vi "Thor8000TCPCommunicator.vi"(0 "EthernetConnection":T1={"IPAddress"="192.168.0.100", "Port"=1234, "Timeout [ms]"=250, "HeaderBytes"=0, "DataBytes"=30}, 5 "ErrorIn":errorcluster, 8 "Data2Write":string=":slot 1;:temp:act? ") -> (14 "Header":string, 16 "DataRead":string=":TEMP:ACT 9.51464272E+000\n", 19 "ErrorOut":errorcluster)   [LabVIEW 2012]
uses:
  WVDNewArchitectureUpdate/WVD_Architecture_Update/TypeDefinitions.llb/TypeDef_WavemeterTCPCluster.ctl
  <vilib>/regexp/Match Regular Expression.xnode
panel:
  # "Currnet Settings:\n++addr 10\n++auto 1\n++eoi 0\n++eos 0\n++eot_enable 0\n++eot_char 0\n++mode 1\n++read_tmo_ms 500\n++savecfg 1\n++ver 01.06.06.00"
  # ":slot 1;:temp:act?"
  # ":slot 2;:ild:act?"
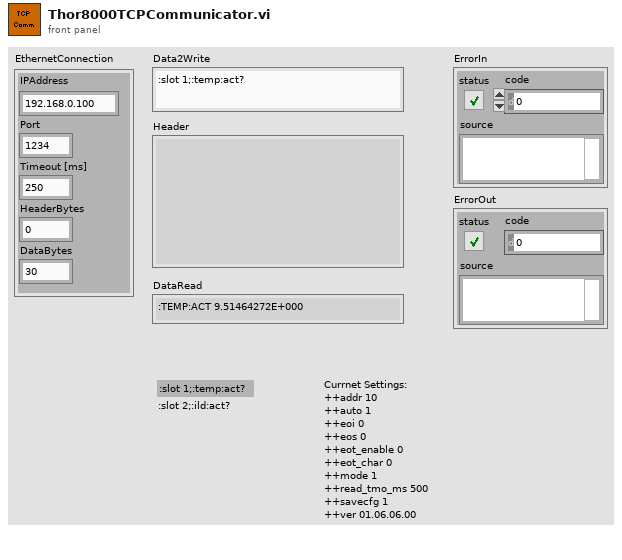
[diagram p1: front panel]
types:
  T1 = typedef "TypeDef_WavemeterTCPCluster.ctl" = cluster{"IPAddress":string, "Port":i16, "Timeout [ms]":i16, "HeaderBytes":i16, "DataBytes":i16}
  T2 = enum16{"Standard", "Buffered", "CRLF", "Immediate"}
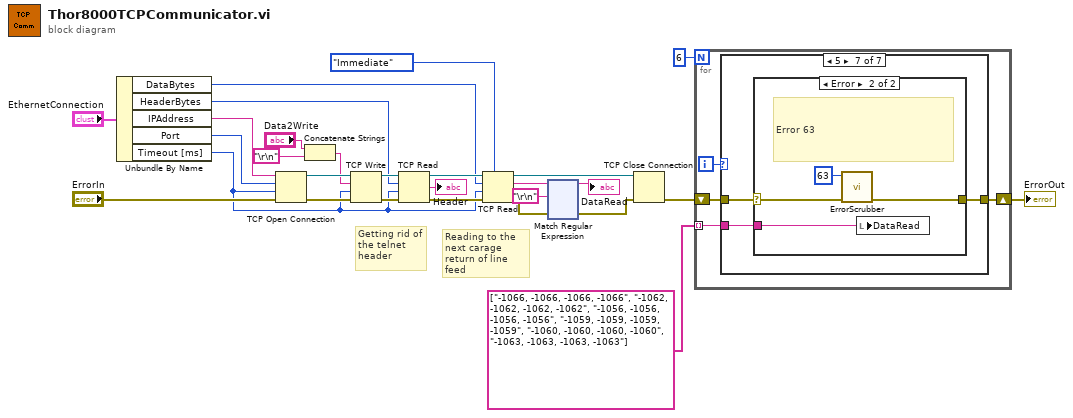
[diagram p0: block diagram]
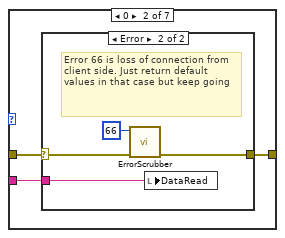
[diagram p3: hidden frame]
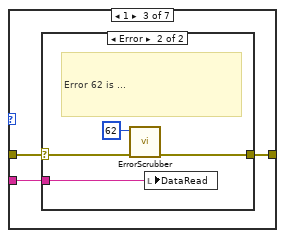
[diagram p5: hidden frame]
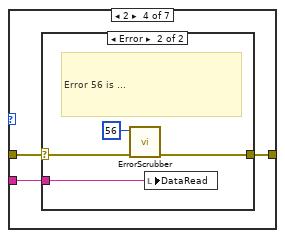
[diagram p7: hidden frame]
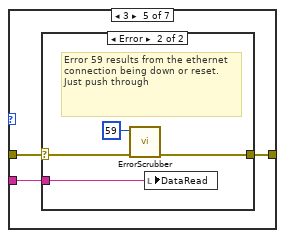
[diagram p9: hidden frame]
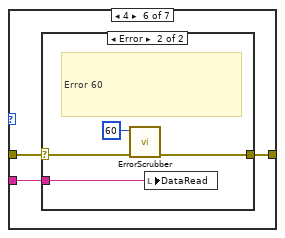
[diagram p11: hidden frame]
diagram:
  # "Reading to the next carage return of line feed"
  # "Getting rid of the telnet header"
  n1 = Unbundle By Name("EthernetConnection") -> ("DataBytes"=w12:i16, "HeaderBytes"=w11:i16, "IPAddress"=w10:string, "Port"=w9:i16, "Timeout [ms]"=w8:i16)
  n2 = TCP Open Connection(address=w10, remote port or service name=w9, timeout ms (60000)=w8, error in (no error)="ErrorIn") -> (connection ID=w27:refnum<k5>, error out=w26:errorcluster)  [unwired: 1 in]
  n3 = Concatenate Strings("Data2Write", "\r\n") -> (w1:string)
  n4 = TCP Write(connection ID=w27, data in=w1, error in (no error)=w26, 9:w8) -> (connection ID out=w23:refnum<k5>, error out=w21:errorcluster)  [unwired: 1 out]
  n5 = TCP Read(connection ID=w23, bytes to read=w11, error in (no error)=w21, 9:w8) -> (connection ID out=w22:refnum<k5>, data out=→"Header":string, error out=w20:errorcluster)  [unwired: 1 in]
  n6 = TCP Read(connection ID=w22, bytes to read=w12, error in (no error)=w20, 7:T2."Immediate" ("mode (standard)"), 9:w8) -> (connection ID out=w25:refnum<k5>, data out=w16:string, error out=w18:errorcluster)
  n7 = xnode "Match Regular Expression"("input string"=w16, "regular expression"="\r\n", "error in"=w18) -> ("before match"=→"DataRead":string, "error out"=w17:errorcluster)  [unwired: 3 in, 3 out]
  n8 = TCP Close Connection(connection ID=w25, error in (no error)=w17) -> (error out=w7:errorcluster)  [unwired: 1 in, 1 out]
  n9 = for {
    N: 6 -> [_]
    shift-right: [w31] -> w6
    shift-left: w7 -> [w32]
    tunnel: string[] ["-1066, -1066, -1066, -1066", "-1062, -1062, -1062, -1062", "-1056, -1056, -1056, -1056", "-1059, -1059, -1059, -1059", "-1060, -1060, -1060, -1060", "-1063, -1063, -1063, -1063"] -> [w29] mode=indexing
    i -> [w30]
    n10 = case shown="5" w30 {
      tunnel: w32 -> [w33 w36 w44 w52 w60 w68 w76]
      tunnel: [w33 w35 w43 w51 w59 w67 w75] -> w31
      tunnel: w29 -> [_ w34 w42 w50 w58 w66 w74]
      frame -1, Default {
      }
      frame 0 {
        n11 = case shown="Error" w36 {
          selector: w36 -> [w37 w40]
          tunnel: [w37 w41] -> w35
          tunnel: w34 -> [_ w38]
          frame No Error {
          }
          frame Error {
            # "Error 66 is loss of connection from client side. Just return default values in that case but keep going"
            n12 = call "ErrorScrubber.vi"("error in (no error)"=w40, "y"=66) -> ("error out"=w41:errorcluster)  [unwired: 8 in, 1 out]
            n13 = local write "DataRead"(w38) -> ()
          }
        }
      }
      frame 1 {
        n14 = case shown="Error" w44 {
          selector: w44 -> [w45 w48]
          tunnel: [w45 w49] -> w43
          tunnel: w42 -> [_ w46]
          frame No Error {
          }
          frame Error {
            # "Error 62 is ..."
            n15 = call "ErrorScrubber.vi"("error in (no error)"=w48, "y"=62) -> ("error out"=w49:errorcluster)  [unwired: 8 in, 1 out]
            n16 = local write "DataRead"(w46) -> ()
          }
        }
      }
      frame 2 {
        n17 = case shown="Error" w52 {
          selector: w52 -> [w53 w56]
          tunnel: [w53 w57] -> w51
          tunnel: w50 -> [_ w54]
          frame No Error {
          }
          frame Error {
            # "Error 56 is ..."
            n18 = call "ErrorScrubber.vi"("error in (no error)"=w56, "y"=56) -> ("error out"=w57:errorcluster)  [unwired: 8 in, 1 out]
            n19 = local write "DataRead"(w54) -> ()
          }
        }
      }
      frame 3 {
        n20 = case shown="Error" w60 {
          selector: w60 -> [w61 w64]
          tunnel: [w61 w65] -> w59
          tunnel: w58 -> [_ w62]
          frame No Error {
          }
          frame Error {
            # "Error 59 results from the ethernet connection being down or reset. Just push through"
            n21 = call "ErrorScrubber.vi"("error in (no error)"=w64, "y"=59) -> ("error out"=w65:errorcluster)  [unwired: 8 in, 1 out]
            n22 = local write "DataRead"(w62) -> ()
          }
        }
      }
      frame 4 {
        n23 = case shown="Error" w68 {
          selector: w68 -> [w69 w72]
          tunnel: [w69 w73] -> w67
          tunnel: w66 -> [_ w70]
          frame No Error {
          }
          frame Error {
            # "Error 60"
            n24 = call "ErrorScrubber.vi"("error in (no error)"=w72, "y"=60) -> ("error out"=w73:errorcluster)  [unwired: 8 in, 1 out]
            n25 = local write "DataRead"(w70) -> ()
          }
        }
      }
      frame 5 {
        n26 = case shown="Error" w76 {
          selector: w76 -> [w77 w80]
          tunnel: [w77 w81] -> w75
          tunnel: w74 -> [_ w78]
          frame No Error {
          }
          frame Error {
            # "Error 63"
            n27 = call "ErrorScrubber.vi"("error in (no error)"=w80, "y"=63) -> ("error out"=w81:errorcluster)  [unwired: 8 in, 1 out]
            n28 = local write "DataRead"(w78) -> ()
          }
        }
      }
    }
  }
  "ErrorOut" <- w6
